vi "Dataset Source 2 Command Types.vi"(10 "Dataset Source":T2=enum."Combined") -> (1 "No Command Types Out":T1[](array[typedef])=[enum."Displacement", enum."Force"], 2 "Command Types":T1[](array[typedef])=[enum."Displacement Command"])   [LabVIEW 2013]
uses:
  Dataset Source.ctl
  Dataset Type.ctl
panel:
  in  "Combined\nNon-Command \nTypes":T1[](array[typedef])=[enum."Displacement", enum."Force"]
  in  "Combined Commands":T1[](array[typedef])=[enum."Displacement Command"]
  in  "Command Types":T1[](array[typedef])=[enum."Displacement Command", enum."Actuator Command"]
  in  "External Sensor Types":T1[](array[typedef])=[enum."LVDT"]
  in  "Non Command Types":T1[](array[typedef])=[enum."Displacement", enum."Force", enum."LVDT", enum."Load Cell"]
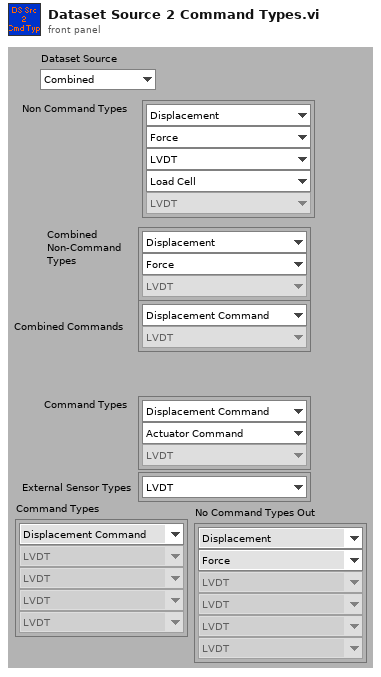
[diagram p1: front panel]
types:
  T1 = typedef "Dataset Type.ctl" = enum16{"LVDT", "Load Cell", "Actuator Command", "Servo Error", "Displacement Command", "Displacement", "Force"}
  T2 = typedef "Dataset Source.ctl" = enum16{"LBCB 1", "LBCB 2", "Combined", "External Sensors"}
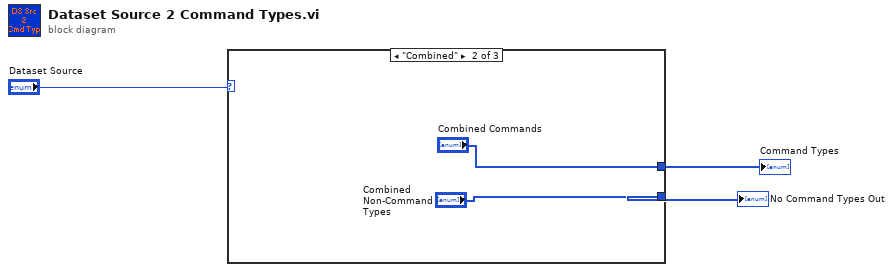
[diagram p0: block diagram]
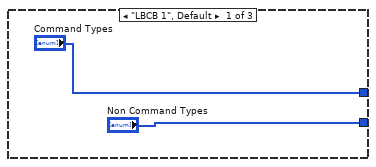
[diagram p2: hidden frame]
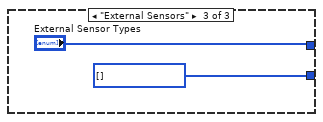
[diagram p3: hidden frame]
diagram:
  n1 = case shown="\"Combined\"" "Dataset Source" {
    tunnel: ["Command Types" "Combined Commands" "External Sensor Types"] -> w2
    tunnel: ["Non Command Types" "Combined\nNon-Command \nTypes" w8] -> w1
    frame "LBCB 1", Default {
    }
    frame "Combined" {
    }
    frame "External Sensors" {
      w8 = T1[] [] items=["LVDT", "Load Cell", "Actuator Command", "Servo Error", "Displacement Command", "Displacement", "Force"] ("Combined Types")
    }
  }
  "Command Types" <- w2
  "No Command Types Out" <- w1
